vi "Label Targets2.vi"(0 "Bottom Clip":dbl, 1 "Valid":bool, 4 "Particle Results":T1(array[cluster]) {"Score" format="%#_3g"; "Pixels"."Rectangle"."Numeric 5" format="%#_3g"; "Pixels"."Rectangle"."Numeric 3" format="%#_3g"; "Pixels"."Rectangle"."Numeric 2" format="%#_3g"; "Pixels"."Rectangle"."Numeric" format="%#_3g"; "Normalized"."Rectangle"."Numeric 5" format="%#_2g"; "Normalized"."Rectangle"."Numeric 3" format="%#_2g"; "Normalized"."Rectangle"."Numeric 2" format="%#_2g"; "Normalized"."Rectangle"."Numeric" format="%#_2g"; "Normalized"."Center"."?" format="%#_3g"; "Normalized"."Center"."?" format="%#_3g"; "Distance (ft)" format="%#_3g"}, 6 "Edges":cluster{"X":sgl, "Y":sgl}[](array[cluster]), 7 "Boiler?":bool, 8 "Line":T2, 9 "Annotate":bool=TRUE, 10 "Results":T4 {"Score" format="%#_3g"; "Pixels"."Rectangle"."Numeric 5" format="%#_3g"; "Pixels"."Rectangle"."Numeric 3" format="%#_3g"; "Pixels"."Rectangle"."Numeric 2" format="%#_3g"; "Pixels"."Rectangle"."Numeric" format="%#_3g"; "Normalized"."Rectangle"."Numeric 5" format="%#_2g"; "Normalized"."Rectangle"."Numeric 3" format="%#_2g"; "Normalized"."Rectangle"."Numeric 2" format="%#_2g"; "Normalized"."Rectangle"."Numeric" format="%#_2g"; "Normalized"."Center"."?" format="%#_3g"; "Normalized"."Center"."?" format="%#_3g"; "Distance (ft)" format="%#_3g"}, 11 "Image in":T3) -> (3 "Image out":T3)   [LabVIEW 2016]
doc: "Draw text values near or on the particle and draws a square around the target stripes.."
uses:
  <vilib>/vision/Image Controls.llb/IMAQ Image.ctl
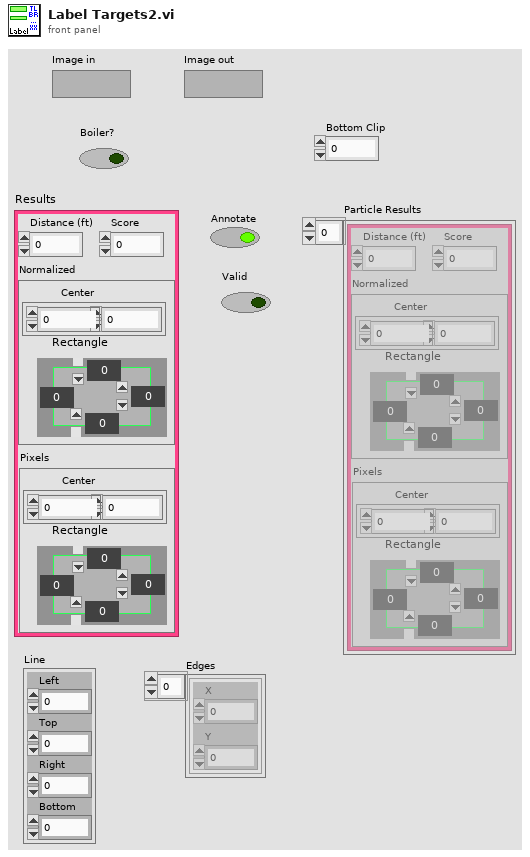
[diagram p1: front panel]
types:
  T1 = cluster{"Distance (ft)":dbl, "Score":dbl, "Normalized":cluster{"Center":cluster{dbl, dbl}, "Rectangle":cluster{"Numeric":dbl, "Numeric 2":dbl, "Numeric 3":dbl, "Numeric 5":dbl}}, "Pixels":cluster{"Center":cluster{dbl, dbl}, "Rectangle":cluster{"Numeric":dbl, "Numeric 2":dbl, "Numeric 3":dbl, "Numeric 5":dbl}}}[]
  T2 = cluster{"Left":dbl, "Top":dbl, "Right":dbl, "Bottom":dbl}
  T3 = typedef "IMAQ Image.ctl" = refnum<image>
  T4 = cluster{"Distance (ft)":dbl, "Score":dbl, "Normalized":cluster{"Center":cluster{dbl, dbl}, "Rectangle":cluster{"Numeric":dbl, "Numeric 2":dbl, "Numeric 3":dbl, "Numeric 5":dbl}}, "Pixels":cluster{"Center":cluster{dbl, dbl}, "Rectangle":cluster{"Numeric":dbl, "Numeric 2":dbl, "Numeric 3":dbl, "Numeric 5":dbl}}}
  T5 = cluster{"Desired Font (Application)":enum16{"User-specified Font", "Application Font", "System Font", "Dialog Font"}, "[User-specified Font]":cluster{"Font Name":string, "Size":i16, "Strikeout?":bool, "Italic?":bool, "Underline?":bool, "Outline?":bool, "Shadow?":bool, "Bold?":bool, "Rotation Angle":dbl}, "Horizontal Alignment":i16, "Vertical Alignment":i16}
  T6 = cluster{"Center":cluster{dbl, dbl}, "Rectangle":cluster{"Numeric":dbl, "Numeric 2":dbl, "Numeric 3":dbl, "Numeric 5":dbl}}
  T7 = cluster{"Numeric":dbl, "Numeric 2":dbl, "Numeric 3":dbl, "Numeric 5":dbl}
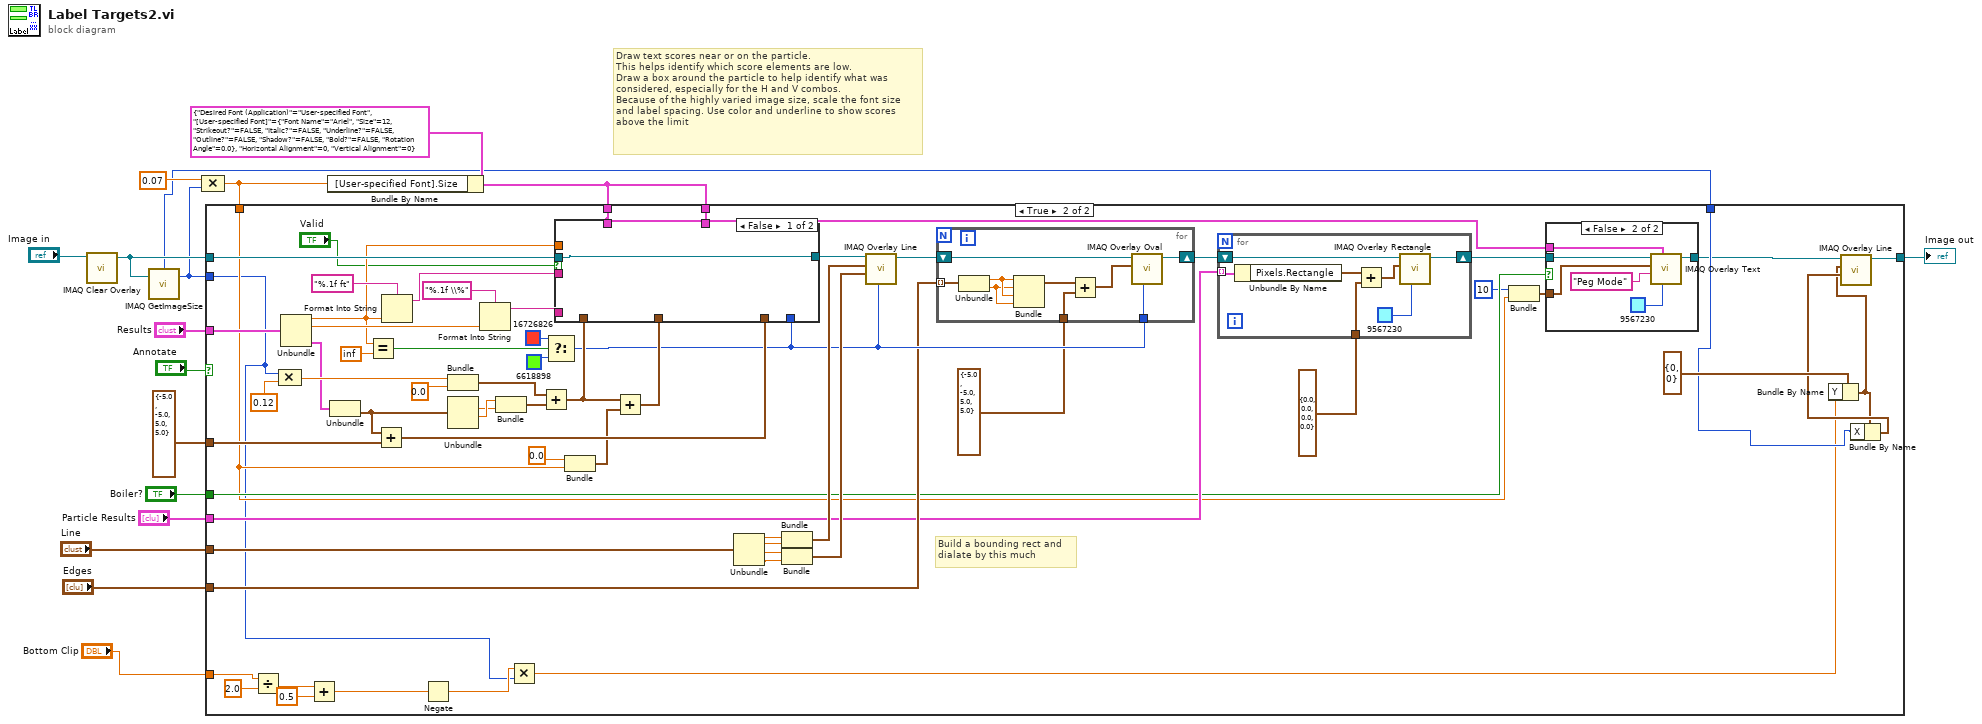
[diagram p0: block diagram]
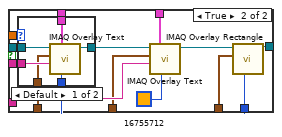
[diagram p3: hidden frame]
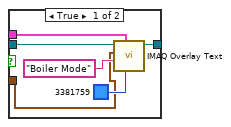
[diagram p5: hidden frame]
diagram:
  # "Draw text scores near or on the particle.\nThis helps identify which score elements are low.\nDraw a box around the particle to help identify what was\nconsidered, especially for the H and V combos.\nBecause of the highly varied image size, scale the font size\nand label spacing. Use color and underline to show scores\nabove the limit"
  n1 = call "IMAQ Clear Overlay"("Image"="Image in") -> ("Image Out"=w12:T3)  [unwired: 2 in, 8 out]
  n2 = call "IMAQ GetImageSize"("Image"=w12) -> ("Y Resolution"=w11:i32, "X Resolution"=w2:i32)  [unwired: 3 in, 1 out]
  n3 = Compound Arithmetic op=MULTIPLY(0.07, w11) -> (w7:dbl)
  n4 = Bundle By Name(cluster=T5 {"Desired Font (Application)"=enum."User-specified Font", "[User-specified Font]"={"Font Name"="Ariel", "Size"=12, "Strikeout?"=FALSE, "Italic?"=FALSE, "Underline?"=FALSE, "Outline?"=FALSE, "Shadow?"=FALSE, "Bold?"=FALSE, "Rotation Angle"=0.0}, "Horizontal Alignment"=0, "Vertical Alignment"=0} ("Font, Size & Style"), "[User-specified Font].Size"=w7) -> (w8:T5)
  n5 = case shown="True" "Annotate" {
    tunnel: [w18 w21] -> w17
    tunnel: "Results" -> [_ w82]
    tunnel: w12 -> [w18 w81]
    tunnel: w8 -> [_ w38]
    tunnel: w11 -> [_ w28]
    tunnel: cluster{dbl, dbl, dbl, dbl} {-5.0, -5.0, 5.0, 5.0} ("output cluster") -> [_ w71]
    tunnel: w8 -> [_ w68]
    tunnel: w7 -> [_ w35]
    tunnel: "Line" -> [_ w55]
    tunnel: "Edges" -> [_ w46]
    tunnel: "Particle Results" -> [_ w41]
    tunnel: "Boiler?" -> [_ w37]
    tunnel: w2 -> [_ w23]
    tunnel: "Bottom Clip" -> [_ w27]
    frame False {
    }
    frame True {
      # "Build a bounding rect and\ndialate by this much"
      n6 = Divide(x=w27, y=2.0) -> (x/y=w30:dbl)
      n7 = Compound Arithmetic op=MULTIPLY(w28, 0.12) -> (w74:dbl)
      n8 = Unbundle(w82) -> ("Distance (ft)"=w44:dbl, "Score"=w67:dbl, "Pixels"=w69:T6)  [unwired: 1 out]
      n9 = Add(x=w30, y=0.5) -> (x+y=w32:dbl)
      n10 = Unbundle(w69) -> ("Rectangle"=w70:T7)  [unwired: 1 out]
      n11 = Equal?(x=w44, y=inf) -> (x = y?=w57:bool)
      n12 = Add(x=w70, y=w71) -> (x+y=w77:cluster{dbl, dbl, dbl, dbl})
      n13 = Format Into String(format string="%.1f ft", w44) -> (resulting string=w72:string)  [unwired: 2 in, 1 out]
      n14 = Negate(x=w32) -> (-x=w33:dbl)
      n15 = Bundle(w74, 0.0) -> (w76:cluster{dbl, dbl})  [unwired: 1 in]
      n16 = Unbundle(w70) -> ("Numeric 2"=w79:dbl, "Numeric 3"=w80:dbl)  [unwired: 2 out]
      n17 = Format Into String(format string="%.1f \\%", w67) -> (resulting string=w65:string)  [unwired: 2 in, 1 out]
      n18 = Bundle("Numeric 3"=w80, "Numeric 2"=w79) -> (w78:cluster{"Numeric 3":dbl, "Numeric 2":dbl})  [unwired: 1 in]
      n19 = Multiply(x=w33, y=w28) -> (x*y=w22:dbl)
      n20 = Add(x=w76, y=w78) -> (x+y=w64:cluster{dbl, dbl})
      n21 = Select(t=u32 16726826 ("Color"), s=w57, f=u32 6618898 ("Color")) -> (s? t:f=w47:u32)
      n22 = Bundle(0.0, w35) -> (w63:cluster{dbl, dbl})  [unwired: 1 in]
      n23 = Add(x=w64, y=w63) -> (x+y=w61:cluster{dbl, dbl})
      n24 = case shown="False" "Valid" {
        tunnel: w81 -> [w83 w97]
        tunnel: w77 -> [_ w96]
        tunnel: w72 -> [_ w95]
        tunnel: w68 -> [_ w92]
        tunnel: w65 -> [_ w90]
        tunnel: w64 -> [_ w89]
        tunnel: w61 -> [_ w88]
        tunnel: w47 -> [_ w87]
        tunnel: w44 -> [_ w86]
        tunnel: [w83 w85] -> w43
        tunnel: w38 -> [_ w84]
        frame False {
        }
        frame True {
          n25 = case shown="Default" w86 {
            tunnel: w97 -> [w103 w104]
            tunnel: w95 -> [w102 _]
            tunnel: w84 -> [w101 _]
            tunnel: [w100 w104] -> w94
            tunnel: w89 -> [w99 _]
            tunnel: w87 -> [w98 _]
            frame Default {
              n26 = call "IMAQ Overlay Text"("Text Color (black)"=w98, "Font, Size & Style"=w101, "String"=w102, "Origin"=w99, "Image"=w103) -> ("Image Out"=w100:T3)  [unwired: 5 in, 1 out]
            }
            frame 0 {
            }
          }
          n27 = call "IMAQ Overlay Text"("Text Color (black)"=u32 16755712 ("Color"), "Font, Size & Style"=w92, "String"=w90, "Origin"=w88, "Image"=w94) -> ("Image Out"=w93:T3)  [unwired: 5 in, 1 out]
          n28 = call "IMAQ Overlay Rectangle"("Color"=w87, "Rectangle"=w96, "Image"=w93) -> ("Image Out"=w85:T3)  [unwired: 7 in, 1 out]
        }
      }
      n29 = Unbundle(w55) -> ("Left"=w54:dbl, "Top"=w53:dbl, "Right"=w52:dbl, "Bottom"=w51:dbl)
      n30 = Bundle("Left"=w54, "Top"=w53) -> (w50:cluster{"Left":dbl, "Top":dbl})  [unwired: 1 in]
      n31 = Bundle("Right"=w52, "Bottom"=w51) -> (w49:cluster{"Right":dbl, "Bottom":dbl})  [unwired: 1 in]
      n32 = call "IMAQ Overlay Line"("Color"=w47, "End Point"=w49, "Start Point"=w50, "Image"=w43) -> ("Image Out"=w48:T3)  [unwired: 6 in, 1 out]
      n33 = for {
        shift-right: [w131] -> w42
        shift-left: w48 -> [w132]
        tunnel: w47 -> [w130]
        tunnel: w46 -> [w128] mode=indexing
        tunnel: cluster{"X":sgl, "Y":sgl, "X":sgl, "Y":sgl} {"X"=-5.0, "Y"=-5.0, "X"=5.0, "Y"=5.0} ("output cluster") -> [w124]
        n34 = Unbundle(w128) -> ("X"=w127:sgl, "Y"=w126:sgl)
        n35 = Bundle("X"=w127, "Y"=w126, "X"=w127, "Y"=w126) -> (w125:cluster{"X":sgl, "Y":sgl, "X":sgl, "Y":sgl})  [unwired: 1 in]
        n36 = Add(x=w125, y=w124) -> (x+y=w129:cluster{"X":sgl, "Y":sgl, "X":sgl, "Y":sgl})
        n37 = call "IMAQ Overlay Oval"("Color"=w130, "Bounding Rectangle"=w129, "Image"=w132) -> ("Image Out"=w131:T3)  [unwired: 7 in, 1 out]
      }
      n38 = for {
        shift-right: [w122] -> w39
        shift-left: w42 -> [w123]
        tunnel: w41 -> [w121] mode=indexing
        tunnel: cluster{"X":sgl, "Y":sgl, "X":sgl, "Y":sgl} {"X"=0.0, "Y"=0.0, "X"=0.0, "Y"=0.0} ("output cluster") -> [w117]
        n39 = Unbundle By Name(w121) -> ("Pixels.Rectangle"=w119:T7)
        n40 = Add(x=w119, y=w117) -> (x+y=w118:cluster{dbl, dbl, dbl, dbl})
        n41 = call "IMAQ Overlay Rectangle"("Color"=u32 9567230, "Rectangle"=w118, "Image"=w123) -> ("Image Out"=w122:T3)  [unwired: 7 in, 1 out]
      }
      n42 = Bundle(10, w35) -> (w34:cluster{i32, dbl})  [unwired: 1 in]
      n43 = case shown="False" w37 {
        tunnel: w39 -> [w110 w116]
        tunnel: [w109 w115] -> w19
        tunnel: w38 -> [w108 w114]
        tunnel: w34 -> [w105 w111]
        frame True {
          n44 = call "IMAQ Overlay Text"("Text Color (black)"=u32 3381759, "Font, Size & Style"=w108, "String"="Boiler Mode", "Origin"=w105, "Image"=w110) -> ("Image Out"=w109:T3)  [unwired: 5 in, 1 out]
        }
        frame False {
          n45 = call "IMAQ Overlay Text"("Text Color (black)"=u32 9567230, "Font, Size & Style"=w114, "String"="Peg Mode", "Origin"=w111, "Image"=w116) -> ("Image Out"=w115:T3)  [unwired: 5 in, 1 out]
        }
      }
      n46 = Bundle By Name(cluster=cluster{"X":i32, "Y":i32} {"X"=0, "Y"=0} ("Start Point"), "Y"=w22) -> (w24:cluster{"X":i32, "Y":i32})
      n47 = Bundle By Name(cluster=w24, "X"=w23) -> (w25:cluster{"X":i32, "Y":i32})
      n48 = call "IMAQ Overlay Line"("End Point"=w25, "Start Point"=w24, "Image"=w19) -> ("Image Out"=w21:T3)  [unwired: 7 in, 1 out]
    }
  }
  "Image out" <- w17
